vi "rslcx_LV2015_L_Over_Frequency_in_CSV_Example.vi"() -> ()   [LabVIEW 2015]
uses:
  <instrlib>/Rohde&Schwarz LCX LCR Meter/Rohde&Schwarz LCX LCR Meter.lvlib
panel:
  out "Voltage":dbl(graph)=0.02583707
  out "Impedance Error":dbl(graph)=3.616
  out "L":dbl(graph)=-inf
  in  "Measurement Impedance Type":i32(ring)=13 caption="Impedance Type (Parallel Capacitance Dissipation Factor)" items=["Parallel Capacitance Dissipation Factor", "Parallel Capacitance Quality Factor", "Parallel Capacitance Conductance", "Parallel Capacitance Parallel Resistance", "Serial Capacitance Dissipation Factor", "Serial Capacitance Quality Factor", "Serial Capacitance Serial Resistance", "Parallel Inductance Dissipation Factor", "Parallel Inductance Quality Factor", "Parallel Inductance Conductance", "Parallel Inductance Parallel Resistance", "Serial Inductance Dissipation Factor", "Serial Inductance Quality Factor", "Serial Inductance Serial Resistance", "Impedance", "Parallel Resistance Susceptance", "Direct Current Resistance", "Mutual Inductance Phase Angle Degree", "Transformer Ratio Phase Angle Degree", "Impedance Phase Angle Degree", "Impedance Phase Angle Rad", "Conductance Susceptance", "Admittance Phase Angle Degree", "Admittance Phase Angle Rad"]
  in  "Measurement Type":i32(ring) caption="Type (L)" items=["L", "C", "R", "T"]
  in  "Frequency Step (Hz)":dbl=50000.0 caption="Frequency (4Hz)" format="%#.9p"
  in  "Frequency End (Hz)":dbl=10000000.0 caption="Frequency (4Hz)" format="%#.9p"
  out "Theta d":dbl(graph)=-6.657536
  in  "Measurement Speed":i32(ring)=1 caption="Measurement Speed (Short)" items=["Short", "Medium", "Long"]
  in  "Frequency Start (Hz)":dbl=500000.0 caption="Frequency (4Hz)" format="%#.9p"
  out "Z":dbl(graph)=2.493273
  out "*IDN? response":string="Rohde&Schwarz,LCX200,3629.8856k03/102063,02.049 007F16294D"
  in  "VISA resource name":refnum<visa-resource-name>="TCPIP::10.102.189.20::hislip0"
  in  "Reset":bool
  in  "ID Query":bool=TRUE
  # "Rohde & Schwarz LCR Meter Measurement Loop Example"
  # "This example shows how to measure several parameters of your test object over frequency.\nPlease note you have to set the instrument to triggered mode (single mode) in order to\nmake sure each measurement value readout is a new one. If you use the function Readxxx(),\na new measurement is triggered, and the instrument returns the measured value.\nFetchxxx() functions only query the previously measured result, hence they save the measurement time.\nNote, that in order to read the Voltage, you have to shortly switch to continuous mode."
  # "Before running, change the VISA resource name to fit your device:\n- For LAN interface use TCPIP::<IP_Address>::INSTR e.g. TCPIP::10.64.0.178::INSTR\n- For USB interface use USB0::0x0AAD::<PID>::<SN>::INSTR e.g. USB0::0x0AAD::0x01D6::101457::INSTR"
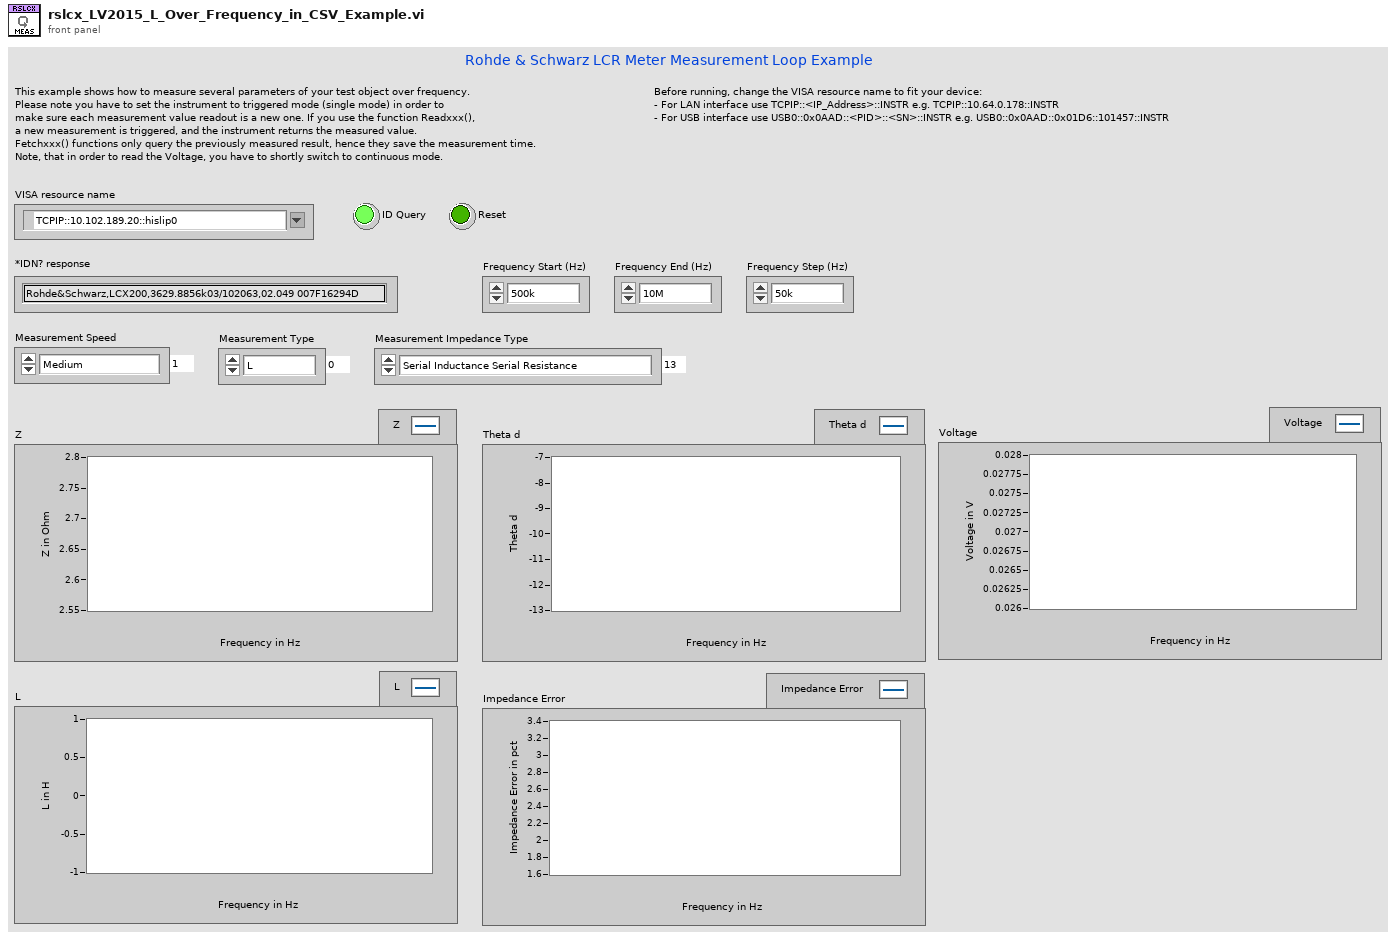
[diagram p1: front panel]
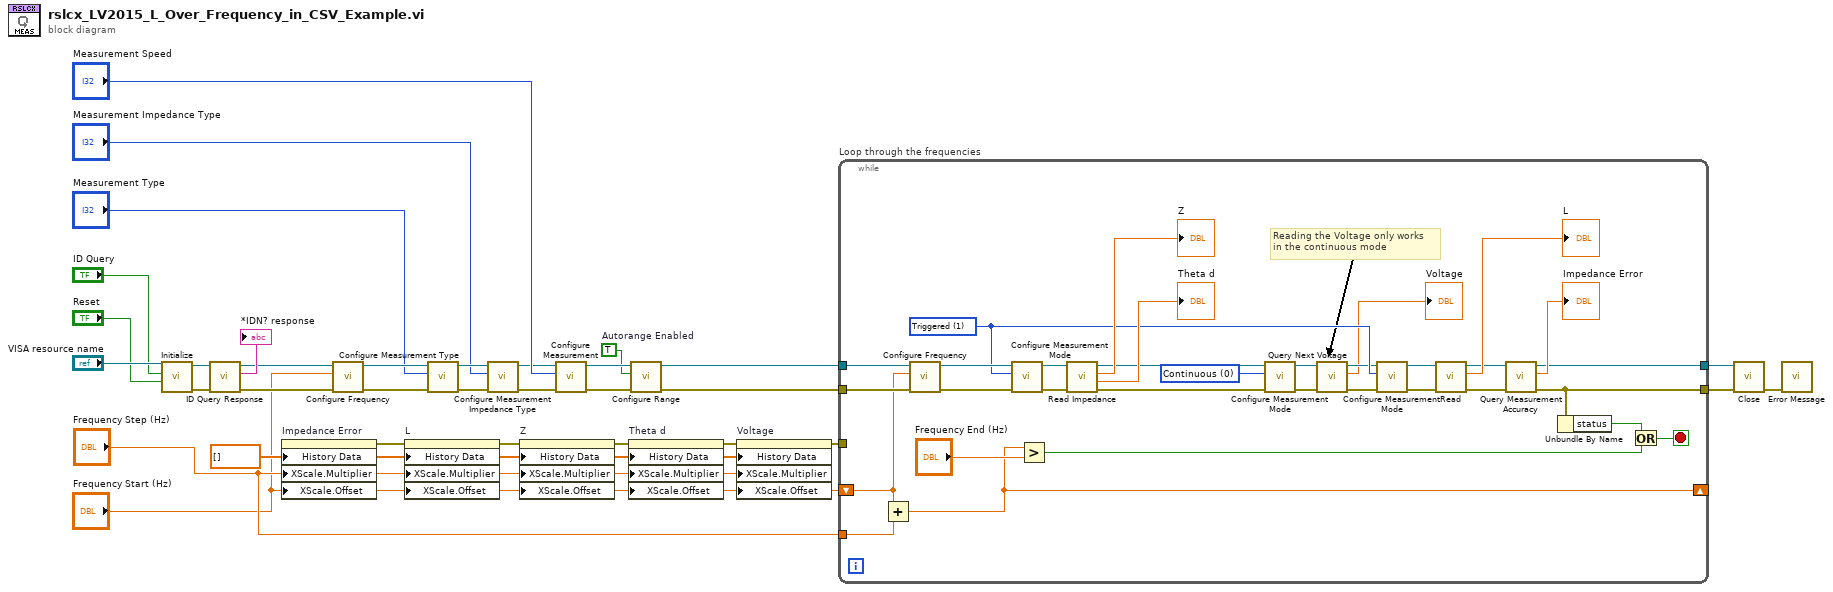
[diagram p0: block diagram]
diagram:
  w3 = dbl[] [] ("History Data")
  w21 = TRUE  # Autorange Enabled
  n1 = call <instrlib>:"Initialize.vi"("Reset (T: Reset)"="Reset", "ID Query (T: Check)"="ID Query", "VISA resource name"="VISA resource name") -> ("error out"=w32:errorcluster, "VISA resource name out"=w31:refnum<visa-resource-name>)  [unwired: 7 in]
  n2 = call <instrlib>:"ID Query Response.vi"("error in (no error)"=w32, "VISA resource name"=w31) -> ("error out"=w26:errorcluster, "ID Query Response"=→"*IDN? response":string, "VISA resource name out"=w25:refnum<visa-resource-name>)  [unwired: 7 in]
  n3 = property on="Impedance Error" class="WFChart (strict)"("History Data"=w3, "XScale.Multiplier"="Frequency Step (Hz)", "XScale.Offset"="Frequency Start (Hz)") -> (error out=w8:errorcluster)  [unwired: 2 in, 1 out]
  n4 = call <instrlib>:"Configure Frequency.vi"("error in (no error)"=w26, "Frequency (4Hz)"="Frequency Start (Hz)", "VISA resource name"=w25) -> ("error out"=w16:errorcluster, "VISA resource name out"=w15:refnum<visa-resource-name>)  [unwired: 7 in]
  n5 = property on="L" class="WFChart (strict)"(error in=w8, "History Data"=w3, "XScale.Multiplier"="Frequency Step (Hz)", "XScale.Offset"="Frequency Start (Hz)") -> (error out=w7:errorcluster)  [unwired: 1 in, 1 out]
  n6 = call <instrlib>:"Configure Measurement Type.vi"("error in (no error)"=w16, "Type (L)"="Measurement Type", "VISA resource name"=w15) -> ("error out"=w13:errorcluster, "VISA resource name out"=w12:refnum<visa-resource-name>)  [unwired: 7 in]
  n7 = call <instrlib>:"Configure Measurement Impedance Type.vi"("error in (no error)"=w13, "Impedance Type (Parallel Capacitance Dissipation Factor)"="Measurement Impedance Type", "VISA resource name"=w12) -> ("error out"=w11:errorcluster, "VISA resource name out"=w10:refnum<visa-resource-name>)  [unwired: 7 in]
  n8 = property on="Z" class="WFChart (strict)"(error in=w7, "History Data"=w3, "XScale.Multiplier"="Frequency Step (Hz)", "XScale.Offset"="Frequency Start (Hz)") -> (error out=w6:errorcluster)  [unwired: 1 in, 1 out]
  n9 = call <instrlib>:"Configure Measurement.vi"("error in (no error)"=w11, "Measurement Speed (Short)"="Measurement Speed", "VISA resource name"=w10) -> ("error out"=w24:errorcluster, "VISA resource name out"=w23:refnum<visa-resource-name>)  [unwired: 7 in]
  n10 = property on="Theta d" class="WFChart (strict)"(error in=w6, "History Data"=w3, "XScale.Multiplier"="Frequency Step (Hz)", "XScale.Offset"="Frequency Start (Hz)") -> (error out=w5:errorcluster)  [unwired: 1 in, 1 out]
  n11 = call <instrlib>:"Configure Range.vi"("error in (no error)"=w24, "Autorange Enabled (On)"=w21, "VISA resource name"=w23) -> ("error out"=w20:errorcluster, "VISA resource name out"=w19:refnum<visa-resource-name>)  [unwired: 7 in]
  n12 = property on="Voltage" class="WFChart (strict)"(error in=w5, "History Data"=w3, "XScale.Multiplier"="Frequency Step (Hz)", "XScale.Offset"="Frequency Start (Hz)") -> (error out=w4:errorcluster)  [unwired: 1 in, 1 out]
  n13 = while "Loop through the frequencies" {
    shift-right: [w54] -> _
    shift-left: "Frequency Start (Hz)" -> [w57]
    tunnel: w20 -> [w65]
    tunnel: w19 -> [w64]
    tunnel: [w38] -> w18
    tunnel: [w36] -> w17
    tunnel: "Frequency Step (Hz)" -> [w35]
    tunnel: w4 -> [_]
    stop <- w56 stop-if-true
    w51 = 0 items=["Continuous", "Triggered"] ("Mode (Continuous)")
    w50 = 1 items=["Continuous", "Triggered"] ("Mode (Continuous)")
    # "Reading the Voltage only works\nin the continuous mode"
    n14 = Add(x=w57, y=w35) -> (x+y=w54:dbl)
    n15 = call <instrlib>:"Configure Frequency.vi"("error in (no error)"=w65, "Frequency (4Hz)"=w57, "VISA resource name"=w64) -> ("error out"=w63:errorcluster, "VISA resource name out"=w62:refnum<visa-resource-name>)  [unwired: 7 in]
    n16 = call <instrlib>:"Configure Measurement Mode.vi"("error in (no error)"=w63, "Mode (Continuous)"=w50, "VISA resource name"=w62) -> ("error out"=w61:errorcluster, "VISA resource name out"=w60:refnum<visa-resource-name>)  [unwired: 7 in]
    n17 = Greater?(x=w54, y="Frequency End (Hz)") -> (0:w52:bool)
    n18 = call <instrlib>:"Read Impedance.vi"("error in (no error)"=w61, "VISA resource name"=w60) -> ("error out"=w49:errorcluster, "Theta d"=→"Theta d":dbl, "Z"=→"Z":dbl, "VISA resource name out"=w48:refnum<visa-resource-name>)  [unwired: 6 in]
    n19 = call <instrlib>:"Configure Measurement Mode.vi"("error in (no error)"=w49, "Mode (Continuous)"=w51, "VISA resource name"=w48) -> ("error out"=w47:errorcluster, "VISA resource name out"=w46:refnum<visa-resource-name>)  [unwired: 7 in]
    n20 = call <instrlib>:"Query Next Voltage.vi"("error in (no error)"=w47, "VISA resource name"=w46) -> ("error out"=w45:errorcluster, "Next Voltage"=→"Voltage":dbl, "VISA resource name out"=w44:refnum<visa-resource-name>)  [unwired: 7 in]
    n21 = call <instrlib>:"Configure Measurement Mode.vi"("error in (no error)"=w45, "Mode (Continuous)"=w50, "VISA resource name"=w44) -> ("error out"=w43:errorcluster, "VISA resource name out"=w42:refnum<visa-resource-name>)  [unwired: 7 in]
    n22 = call <instrlib>:"Read.vi"("error in (no error)"=w43, "VISA resource name"=w42) -> ("error out"=w40:errorcluster, "Z"=→"L":dbl, "VISA resource name out"=w39:refnum<visa-resource-name>)  [unwired: 6 in, 1 out]
    n23 = call <instrlib>:"Query Measurement Accuracy.vi"("error in (no error)"=w40, "VISA resource name"=w39) -> ("error out"=w38:errorcluster, "Z"=→"Impedance Error":dbl, "VISA resource name out"=w36:refnum<visa-resource-name>)  [unwired: 6 in, 1 out]
    n24 = Unbundle By Name(w38) -> ("status"=w53:bool)
    n25 = Or(x=w53, y=w52) -> (x .or. y?=w56:bool)
  }
  n26 = call <instrlib>:"Close.vi"("error in (no error)"=w18, "VISA resource name"=w17) -> ("error out"=w30:errorcluster)  [unwired: 9 in]
  n27 = call <instrlib>:"Error Message.vi"("error in (no error)"=w30) -> ()  [unwired: 10 in, 5 out]
